vi "Mavg method.vi"(4 "Encoder Position":i16, 5 "Tick Count (usec)":i16, 6 "D_d_pre":fxp<+/-,49,33>, 7 "x >= y ?":bool, 8 "Array2_pre":i32[](array[numeric])=[0, 0, 0, 0, 0, 0, 0, 0, 0, 0, 0, 0, 0, 0, 0, 0, 0, 0, 0, 0, 0, 0, 0, 0, 0], 9 "element2":i16, 10 "Array1_pre":i32[](array[numeric])=[0, 0, 0, 0, 0, 0, 0, 0, 0, 0, 0, 0, 0, 0, 0, 0, 0, 0, 0, 0, 0, 0, 0, 0, 0], 11 "element1":i16) -> (0 "D_d":fxp<+/-,49,33>, 1 "Array2":i32[](array[numeric]), 2 "Array1":i32[](array[numeric]), 3 "omega":fxp<+/-,64,35>)   [LabVIEW 2014]
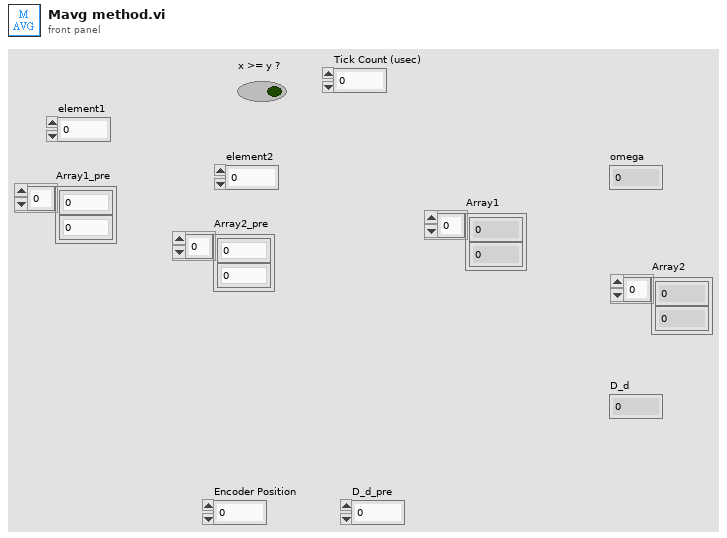
[diagram p1: front panel]
types:
  T1 = cluster{"Array2_pre[0]":i32, "Array2_pre[1]":i32, "Array2_pre[2]":i32, "Array2_pre[3]":i32, "Array2_pre[4]":i32, "Array2_pre[5]":i32, "Array2_pre[6]":i32, "Array2_pre[7]":i32, "Array2_pre[8]":i32, "Array2_pre[9]":i32, "Array2_pre[10]":i32, "Array2_pre[11]":i32, "Array2_pre[12]":i32, "Array2_pre[13]":i32, "Array2_pre[14]":i32, "Array2_pre[15]":i32, "Array2_pre[16]":i32, "Array2_pre[17]":i32, "Array2_pre[18]":i32, "Array2_pre[19]":i32, "Array2_pre[20]":i32, "Array2_pre[21]":i32, "Array2_pre[22]":i32, "Array2_pre[23]":i32, "Array2_pre[24]":i32}
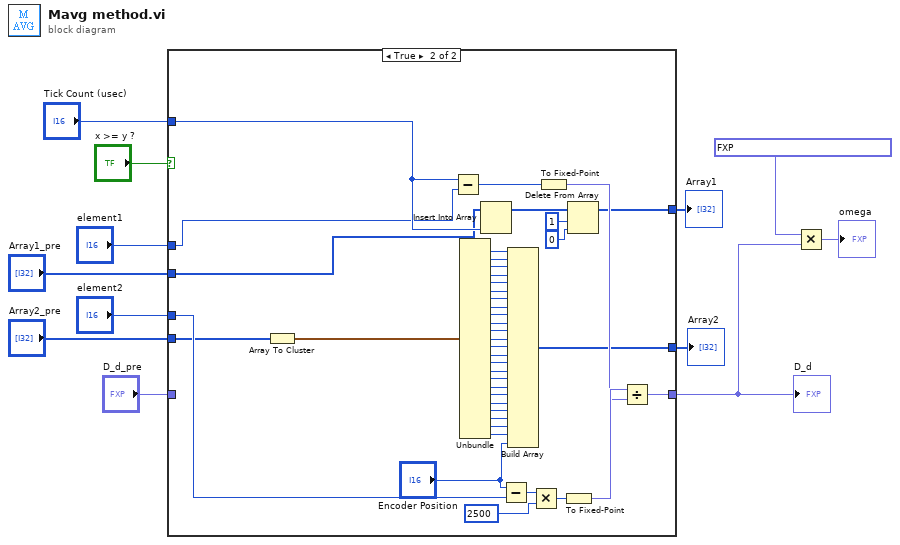
[diagram p0: block diagram]
diagram:
  n1 = case shown="True" "x >= y ?" {
    tunnel: "Tick Count (usec)" -> [_ w54]
    tunnel: "element1" -> [_ w53]
    tunnel: "element2" -> [_ w46]
    tunnel: "Array1_pre" -> [w15 w52]
    tunnel: "Array2_pre" -> [w14 w43]
    tunnel: [w13 w45] -> w4
    tunnel: [w14 w17] -> w1
    tunnel: [w15 w44] -> w2
    tunnel: "D_d_pre" -> [w13 _]
    frame False {
    }
    frame True {
      n2 = Array To Cluster(array=w43) -> (cluster=w42:T1)
      n3 = Subtract(x=w54, y=w53) -> (x-y=w55:i16)
      n4 = Unbundle(w42) -> ("Array2_pre[1]"=w18:i32, "Array2_pre[2]"=w19:i32, "Array2_pre[3]"=w20:i32, "Array2_pre[4]"=w21:i32, "Array2_pre[5]"=w22:i32, "Array2_pre[6]"=w23:i32, "Array2_pre[7]"=w24:i32, "Array2_pre[8]"=w25:i32, "Array2_pre[9]"=w26:i32, "Array2_pre[10]"=w27:i32, "Array2_pre[11]"=w28:i32, "Array2_pre[12]"=w29:i32, "Array2_pre[13]"=w30:i32, "Array2_pre[14]"=w31:i32, "Array2_pre[15]"=w32:i32, "Array2_pre[16]"=w33:i32, "Array2_pre[17]"=w34:i32, "Array2_pre[18]"=w35:i32, "Array2_pre[19]"=w36:i32, "Array2_pre[20]"=w37:i32, "Array2_pre[21]"=w38:i32, "Array2_pre[22]"=w39:i32, "Array2_pre[23]"=w40:i32, "Array2_pre[24]"=w41:i32)  [unwired: 1 out]
      n5 = Insert Into Array(array=w52, new element=w54) -> (w57:i32[])  [unwired: 1 in]
      n6 = Subtract(x="Encoder Position", y=w46) -> (x-y=w51:i16)
      n7 = Build Array(w18, w19, w20, w21, w22, w23, w24, w25, w26, w27, w28, w29, w30, w31, w32, w33, w34, w35, w36, w37, w38, w39, w40, w41, "Encoder Position") -> (w17:i32[])
      n8 = Multiply(x=w51, y=2500) -> (x*y=w49:i32)
      n9 = To Fixed-Point(number=w55) -> (fixed-point=w47:fxp<+/-,16,16>)  [unwired: 1 in]
      n10 = To Fixed-Point(number=w49) -> (fixed-point=w48:fxp<+/-,32,32>)  [unwired: 1 in]
      n11 = Delete From Array(array=w57, length=1, index=0) -> (array with subset deleted=w44:i32[])  [unwired: 1 out]
      n12 = Divide(x=w48, y=w47) -> (x/y=w45:fxp<+/-,49,33>)
    }
  }
  "D_d" <- w4
  "Array1" <- w2
  "Array2" <- w1
  n13 = Multiply(x=fxp<+/-,27,3> 3.1415926218032837, y=w4) -> (x*y=→"omega":fxp<+/-,64,35>)
